vi "Auto Calibrate.vi"(8 "error in (no error)":errorcluster, 11 "Yokogawa AQ6370D in":refnum<class "Yokogawa AQ6370D.lvclass">) -> (0 "error out":errorcluster, 3 "Yokogawa AQ6370D out":refnum<class "Yokogawa AQ6370D.lvclass">)   [LabVIEW 2018, in "Yokogawa AQ6370D.lvlib" / "Yokogawa AQ6370D.lvclass"]
uses:
  Yokogawa AQ6370D.lvclass
  builds/OSA.lvlibp/Optical Spectrum Analyzer.lvclass
  C:/Projects/LabVIEW/In-Progress/Chetan Malpure/Optical Spectrum Analyzer/builds/OSA.lvlibp/Optical Spectrum Analyzer.lvclass
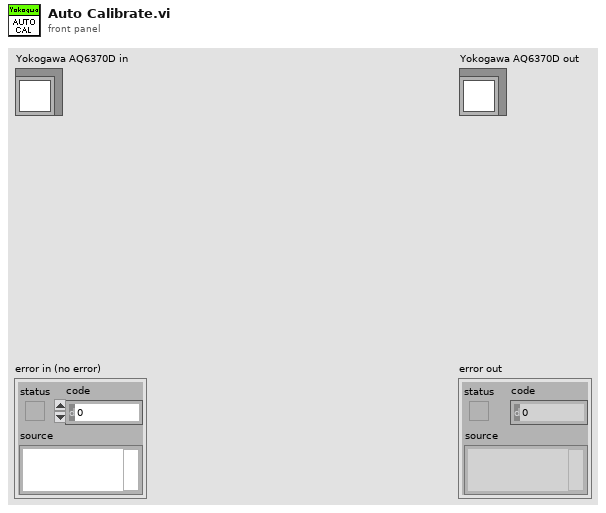
[diagram p1: front panel]
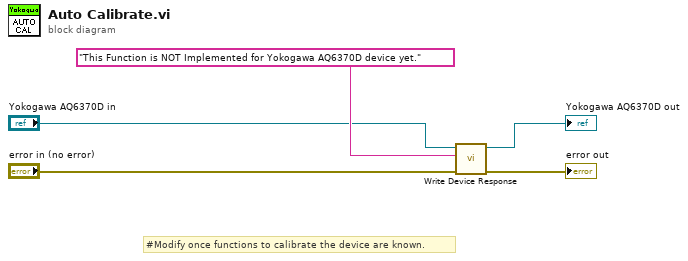
[diagram p0: block diagram]
diagram:
  # "#Modify once functions to calibrate the device are known."
  n1 = call "Write Device Response.vi"("error in (no error)"="error in (no error)", "Device Response"="This Function is NOT Implemented for Yokogawa AQ6370D device yet.", "Optical Spectrum Analyzer in"="Yokogawa AQ6370D in") -> ("error out"=→"error out":errorcluster, "Optical Spectrum Analyzer out"=→"Yokogawa AQ6370D out":refnum<class "Yokogawa AQ6370D.lvclass">)  [unwired: 7 in]
